vi "Read.vi"(8 "error in (no error)":errorcluster, 11 "Boolean in":refnum<class "conc_SharedVar_I8.lvclass">) -> (0 "error out":errorcluster, 2 "Numeric":i8, 3 "Boolean out":refnum<class "conc_SharedVar_I8.lvclass">)   [LabVIEW 2021, in "conc_SharedVar_I8.lvclass"]
doc: "LVabs_Shared Variable 1.0.0.2\nTim - TSA\nCopyright (c) 2024, TSA"
uses:
  conc_SharedVar_I8.lvclass
  conc_SharedVar_I8.lvclass/conc_SharedVar_I8.ctl
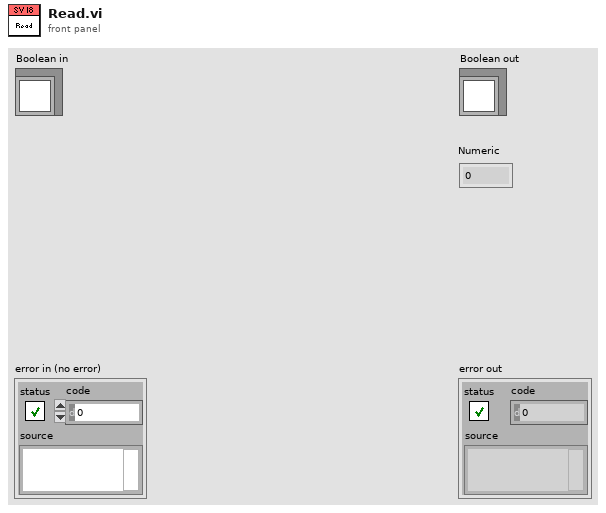
[diagram p1: front panel]
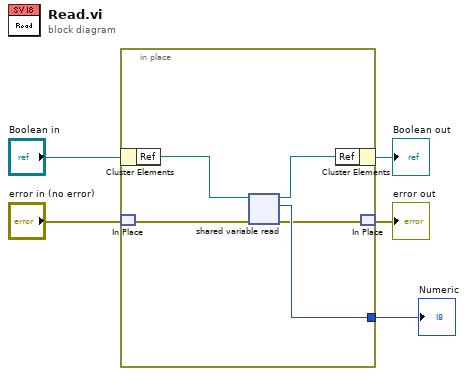
[diagram p0: block diagram]
diagram:
  n1 = in-place {
    in-place-border: [w10] -> w5
    n2 = in-place-cluster #1("Boolean in") -> ("Ref"=w9:refnum<k21>)
    n3 = in-place-match #2("error in (no error)") -> (w7:errorcluster)
    n4 = shared-variable-read(w9, w7) -> (w8:refnum<k21>, w6:errorcluster, w10:i8)  [unwired: 1 out]
    n5 = in-place-cluster #1("Ref"=w8) -> (→"Boolean out":refnum<class "conc_SharedVar_I8.lvclass">)
    n6 = in-place-match #2(w6) -> (→"error out":errorcluster)
  }
  "Numeric" <- w5
